vi "Connection Monitor - Loop.vi"(8 "error in (no error)":errorcluster, 11 "RemoteControl.STM in":refnum<class "RemoteControl.STM.lvclass">) -> (0 "error out":errorcluster, 3 "RemoteControl.STM out":refnum<class "RemoteControl.STM.lvclass">)   [LabVIEW 2019, in "RemoteControl.STM.lvclass"]
uses:
  RemoteControl.STM.lvclass
  <vilib>/NI/STM/Connection Manager/TCP/TCP Connection Method.ctl
  <vilib>/NI/STM/TCP/Write Meta Data (TCP Ref).vi
  <vilib>/NI/STM/TCP/Write Meta Data (TCP Clst).vi
  <userlib>/_OpenG.lib/error/error.llb/Filter Error Codes (Array)__ogtk.vi
  <vilib>/NI/STM/NI STM.lvlib
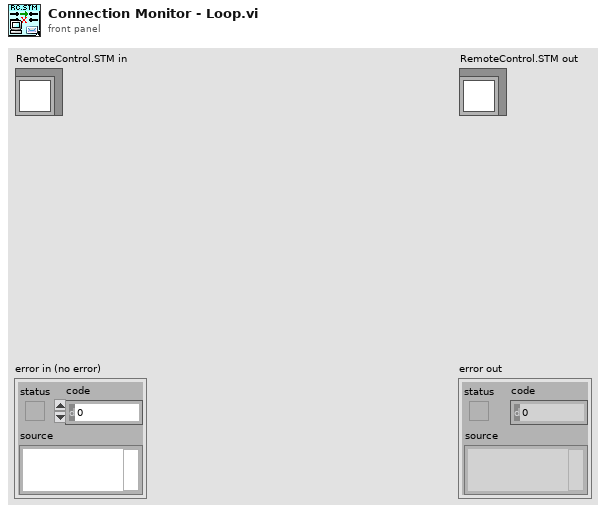
[diagram p1: front panel]
types:
  T1 = typedef "NI STM.lvlib/TCP Connection Method.ctl" = enum16{"Initialize", "Add Connection", "Set Properties", "Get Connection(s)", "Remove Connection", "Remove All Connections", "Get Connection Count"}
  T2 = typedef "NI STM.lvlib/TCP Connection Info.ctl" = cluster{"connection ID":refnum<k5>, "meta data":T3[]}
  T3 = typedef "NI STM.lvlib/MetaDataElement.ctl" = string
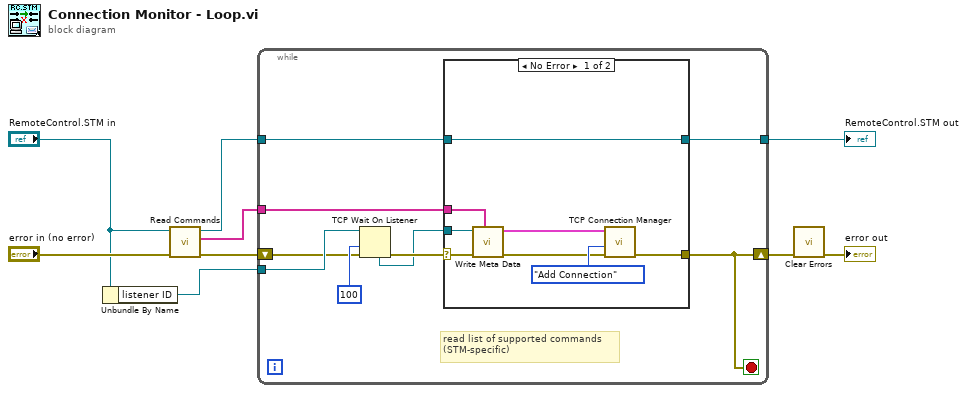
[diagram p0: block diagram]
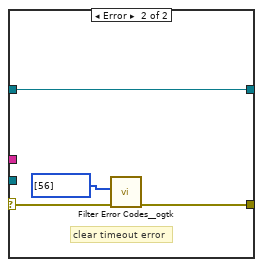
[diagram p2: hidden frame]
diagram:
  n1 = Unbundle By Name("RemoteControl.STM in") -> ("listener ID"=w5:refnum<k5>)
  n2 = call-dynamic "Read Commands.vi"("error in (no error)"="error in (no error)", "RemoteControl in"="RemoteControl.STM in") -> ("error out"=w7:errorcluster, "Commands"=w1:string[], "RemoteControl out"=w2:refnum<class "RemoteControl.STM.lvclass">)  [unwired: 7 in]
  n3 = while {
    shift-right: [w15] -> w9
    shift-left: w7 -> [w11]
    tunnel: w5 -> [w14]
    tunnel: w1 -> [w13]
    tunnel: w2 -> [w12]
    tunnel: [w16] -> w8
    stop <- w15 stop-if-true
    # "read list of supported commands\n(STM-specific)"
    n4 = TCP Wait On Listener(8:w11, 9:100 ("timeout ms (wait forever: -1)"), 11:w14) -> (0:w18:errorcluster, 4:w10:refnum<k5>)  [unwired: 1 in, 3 out]
    n5 = case shown="No Error" w18 {
      selector: w18 -> [w19 w29]
      tunnel: w10 -> [w26 _]
      tunnel: [w23 w28] -> w15
      tunnel: [w20 w27] -> w16
      tunnel: w12 -> [w20 w27]
      tunnel: w13 -> [w21 _]
      frame No Error {
        n6 = call-poly <vilib>:"Write Meta Data.vi"("meta data"=w21, "error in"=w19, "connection ID"=w26) -> ("error out"=w24:errorcluster, "connection info out"=w22:T2)  [unwired: 7 in]
        n7 = call <vilib>:"TCP Connection Manager.vi"("error in"=w24, "method"=TCP_Connection_Method."Add Connection", "connection in"=w22) -> ("error out"=w23:errorcluster)  [unwired: 3 in, 5 out]
      }
      frame Error {
        # "clear timeout error"
        n8 = call-poly <userlib>:"Filter Error Codes__ogtk.vi"("Error In"=w29, "Error Codes to Filter"=i32[] [56]) -> ("Error Out"=w28:errorcluster)  [unwired: 7 in, 2 out]
      }
    }
  }
  "RemoteControl.STM out" <- w8
  n9 = call <vilib>:"Clear Errors.vi"("error in (no error)"=w9) -> ("error out"=→"error out":errorcluster)  [unwired: 5 in, 1 out]
